vi "FilterEvent.vi"() -> ()   [LabVIEW 2020]
panel:
  in  "Stop":bool
  in  "Control":u16
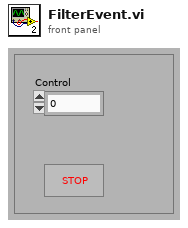
[diagram p1: front panel]
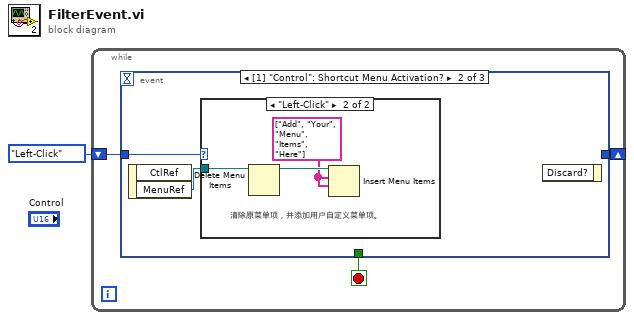
[diagram p0: block diagram]
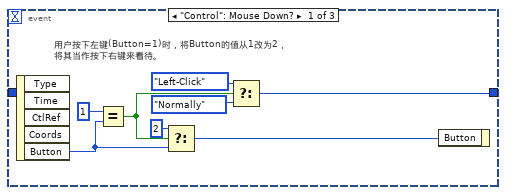
[diagram p2: hidden frame]
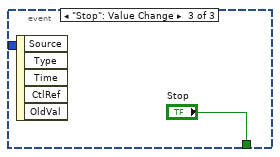
[diagram p4: hidden frame]
diagram:
  n1 = while {
    shift-right: [w3] -> _
    shift-left: enum16{"Normally", "Left-Click"}."Left-Click" ("Enum") -> [w2]
    stop <- w4 stop-if-true
    n2 = event shown="[1] \"Control\": Shortcut Menu Activation?" {
      selector: _ -> [_ _ _]
      dyn-events: _ -> [_ _ _]
      timeout: _ -> [_ _ _]
      tunnel: [_ _ "Stop"] -> w4
      tunnel: [w12 _ _] -> w3
      tunnel: w2 -> [_ w14 _]
      event "Control": Mouse Down? {
        # "用户按下左键(Button=1)时，将Button的值从1改为2，\n将其当作按下右键来看待。"
        n3 = event-data() -> ("Button"=w7:u16)  [unwired: 5 out]
        n4 = Equal?(x=u16 1, y=w7) -> (x = y?=w9:bool)
        n5 = Select(t=u16 2, s=w9, f=w7) -> (s? t:f=w11:u16)
        n6 = Select(t=enum16{"Normally", "Left-Click"}."Left-Click" ("Enum"), s=w9, f=enum16{"Normally", "Left-Click"}."Normally" ("Enum")) -> (s? t:f=w12:enum16{"Normally", "Left-Click"})
        n7 = event-data("Button"=w11) -> ()  [unwired: 1 in, 1 out]
      }
      event "Control": Shortcut Menu Activation? {
        n8 = event-data() -> ("MenuRef"=w13:refnum<k9>)  [unwired: 2 out]
        n9 = case shown="\"Left-Click\"" w14 {
          tunnel: w13 -> [_ w17]
          frame "Normally", Default {
            # "不对菜单进行修改"
          }
          frame "Left-Click" {
            w15 = string[] ["Add", "Your", "Menu", "Items", "Here"]
            # "清除原菜单项，并添加用户自定义菜单项。"
            n10 = Delete Menu Items(9:w17) -> (3:w16:refnum<k9>)  [unwired: 1 in, 3 out]
            n11 = Insert Menu Items(7:w15, 8:w15, 9:w16) -> ()  [unwired: 1 in, 5 out]
          }
        }
        n12 = event-data() -> ()  [unwired: 1 in, 2 out]
      }
      event "Stop": Value Change {
        n13 = event-data() -> ()  [unwired: 6 out]
      }
    }
  }
